vi "SetClockHW.vi"(8 "error in (no error)":errorcluster, 11 "BME_DG_G08 in":refnum<class "BME_DG_G08.lvclass">) -> (0 "error out":errorcluster, 3 "BME_DG_G08 out":refnum<class "BME_DG_G08.lvclass">)   [LabVIEW 2009, in "POLARIS BME DG.lvlib" / "BME_DG_G08.lvclass"]
uses:
  BME_DG_G08.lvclass
  BME_DG_G08.lvclass/BME_DG_G08.ctl
  POLARIS BME DG.lvlib
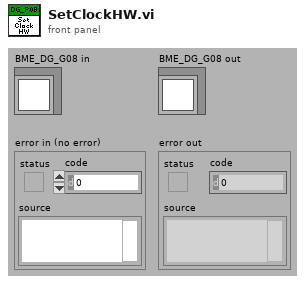
[diagram p1: front panel]
types:
  T1 = typedef "POLARIS BME DG.lvlib/ClockSource.ctl" = i32
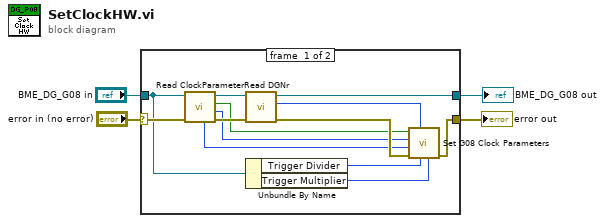
[diagram p0: block diagram]
diagram:
  n1 = case shown="No Error" "error in (no error)" {
    selector: "error in (no error)" -> [w12 w18]
    tunnel: [w17 w18] -> w3
    tunnel: [w15 w19] -> w2
    tunnel: "BME_DG_G08 in" -> [w7 w19]
    frame #0 {
      n2 = call-dynamic "Read ClockParameter.vi"("error in (no error)"=w12, "BME_DG_Base in"=w7) -> ("error out"=w13:errorcluster, "PrescalerCrystalOsc"=w9:u32, "ClockEnable"=w10:bool, "BME_DG_Base out"=w16:refnum<class "BME_DG_G08.lvclass">, "ClockSource"=w8:T1)  [unwired: 5 in]
      n3 = call-dynamic "Read DGNr.vi"("error in (no error)"=w13, "BME_DG_Base in"=w16) -> ("error out"=w11:errorcluster, "DGNr"=w14:i32, "BME_DG_Base out"=w15:refnum<class "BME_DG_G08.lvclass">)  [unwired: 7 in]
      n4 = Unbundle By Name(w7) -> ("Trigger Divider"=w6:u32, "Trigger Multiplier"=w5:u32)
      n5 = call "Set G08 Clock Parameters.vi"("Trigger Multiplier"=w5, "Trigger Divider"=w6, "DG Number"=w14, "error in (no error)"=w11, "Clock Source"=w8, "Ocillator Divider"=w9, "Clock Enable"=w10) -> ("error out"=w17:errorcluster)  [unwired: 4 in]
    }
    frame #1 {
    }
  }
  "error out" <- w3
  "BME_DG_G08 out" <- w2
